vi "EINDE3.vi"() -> ()   [LabVIEW 2018]
uses:
  Kleuren- en afstandsensor/FSM States.ctl
  FSM States Project TOTAAL.ctl
panel:
  out "Achteruit":i32
  out "Timerrijden":i32
  out "Initial State":T1=enum."MOVE DOWNWARDS"
  out "Tussentijd":i32
  out "Timer":i32
  out "The End":bool
  in  "stop 3":bool
  in  "ON/OFF Grijper":bool
  in  "stop":bool
  in  "Aantal Witte blokjes":dbl
  in  "Aantal rode blokjes":dbl
  in  "Aantal Zwarte blokjes":dbl
  in  "LED aansturen":bool[](array[boolean])
  out "Current State":T1
  out "Motor":bool[](array[boolean])
  out "State to recover from":T1=enum."Stilstaan"
  in  "EMERGENCY":bool
  in  "Teller wit":dbl
  in  "Teller Rood":dbl
  in  "Teller zwart":dbl
  out "Wit":bool
  out "Zwart":bool
  out "Rood":bool
  in  "Kleurmaken":bool
  out "Kleuren veranderen":T2
  out "Analoge in":dbl[](array[numeric]) format="%0.2f"
  out "Afstand":bool
  # "INPUT"
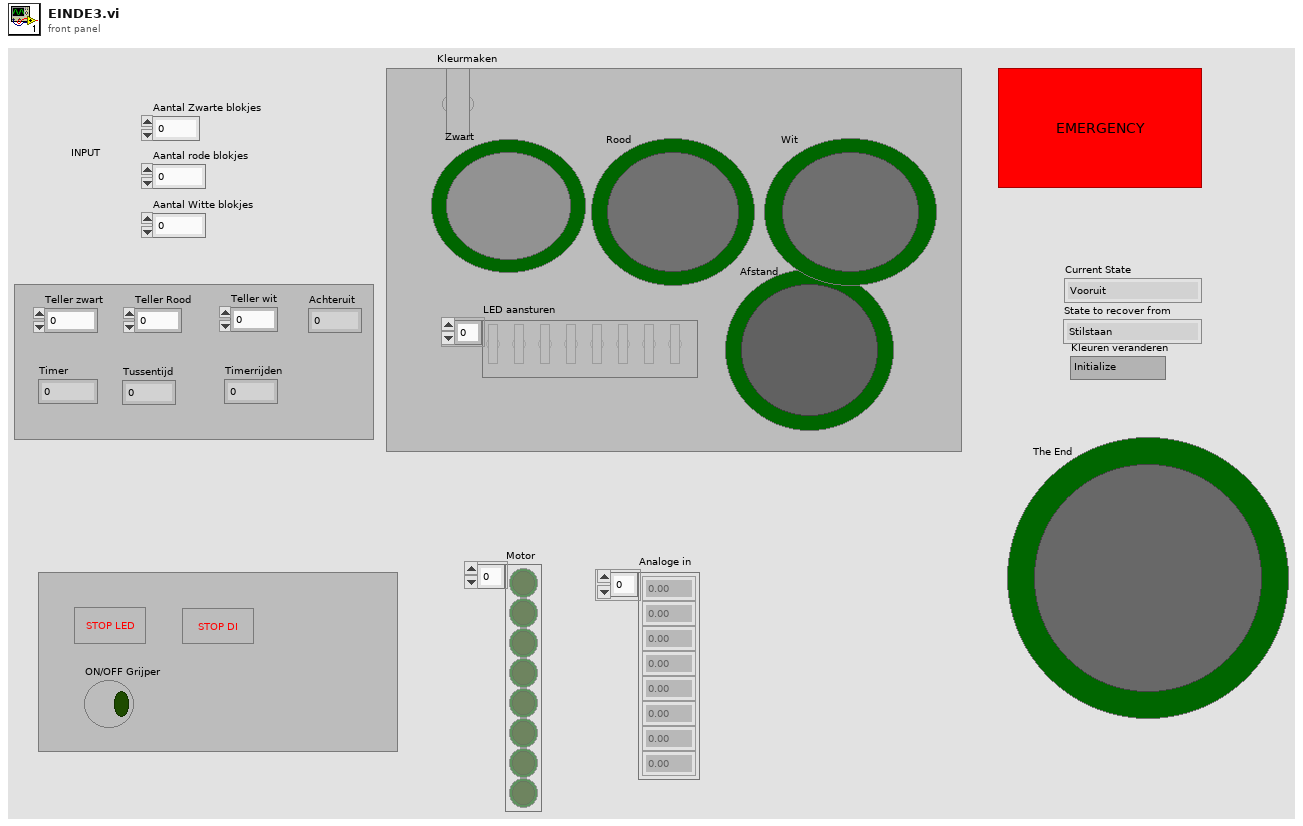
[diagram p1: front panel]
types:
  T1 = typedef "FSM States Project TOTAAL.ctl" = enum16{"Vooruit", "Achteruit", "Stilstaan", "EMERGENCY", "MOVE DOWNWARDS", "GRAB", "MOVE UPWARDS", "ROTATE", "DROP", "RETURN", "Stop "}
  T2 = typedef "FSM States.ctl" = enum16{"Initialize", "ROOD", "GROEN ", "Blauw "}
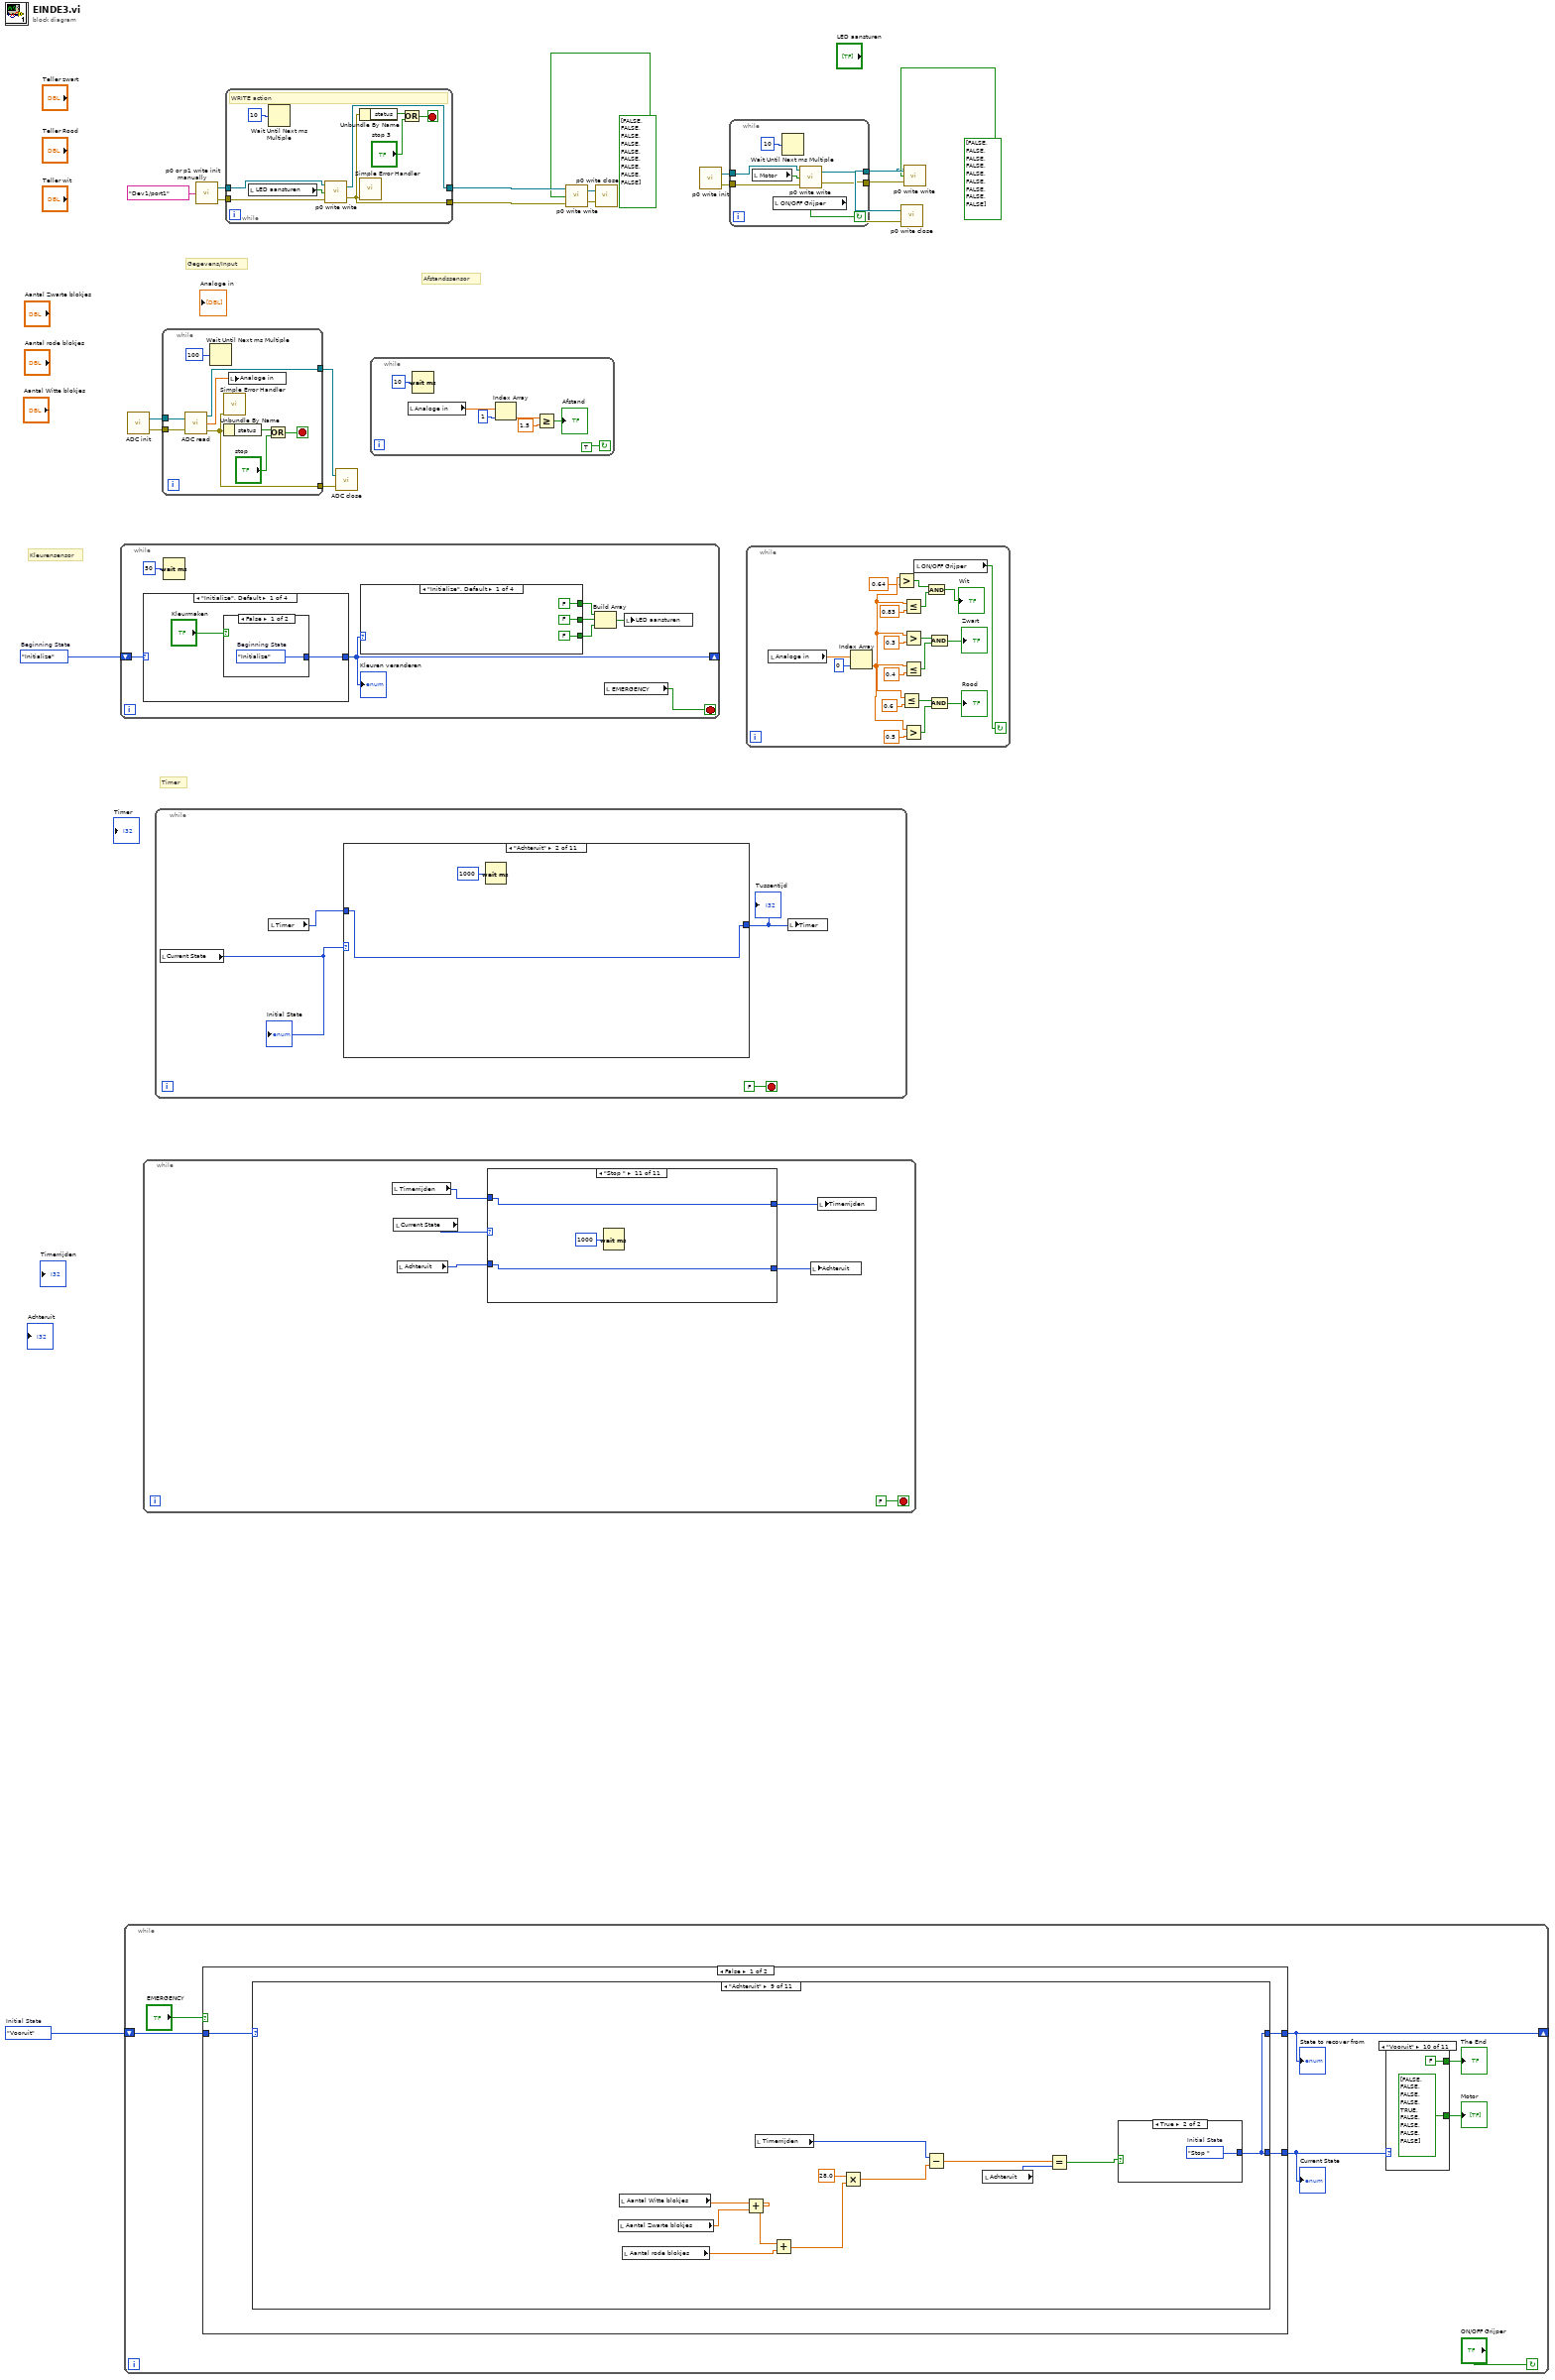
[diagram p0: block diagram]
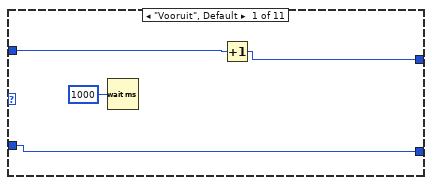
[diagram p2: hidden frame]
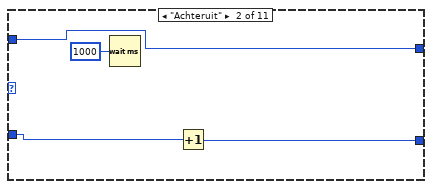
[diagram p3: hidden frame]
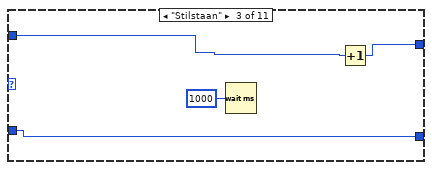
[diagram p4: hidden frame]
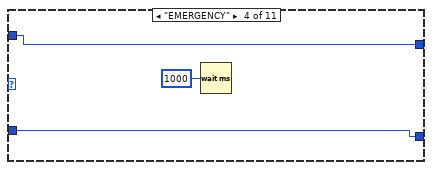
[diagram p5: hidden frame]
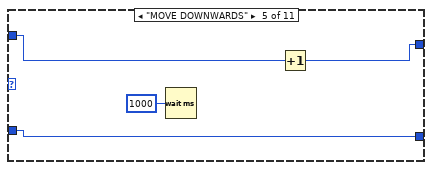
[diagram p6: hidden frame]
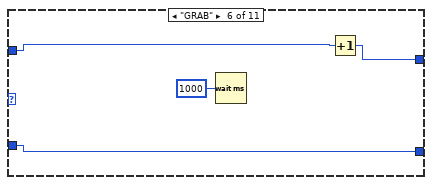
[diagram p7: hidden frame]
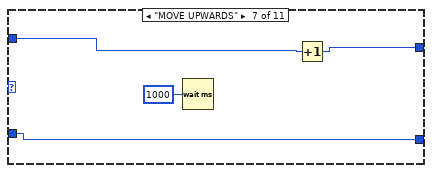
[diagram p8: hidden frame]
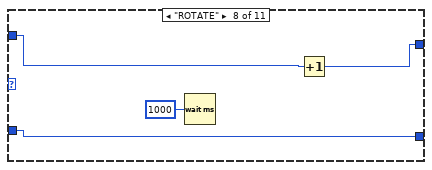
[diagram p9: hidden frame]
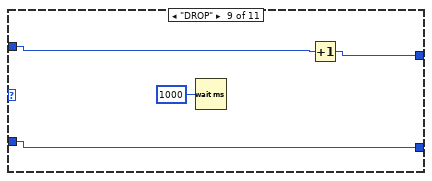
[diagram p10: hidden frame]
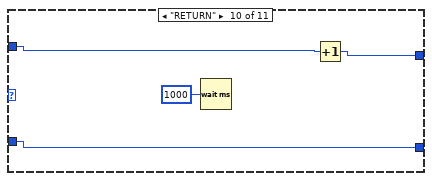
[diagram p11: hidden frame]
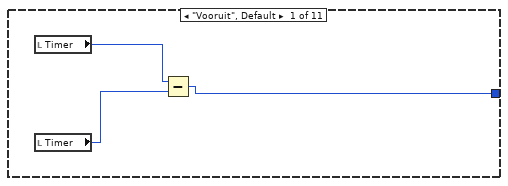
[diagram p12: hidden frame]
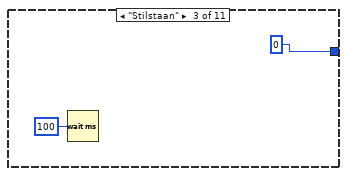
[diagram p13: hidden frame]
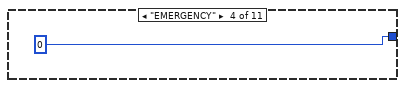
[diagram p14: hidden frame]
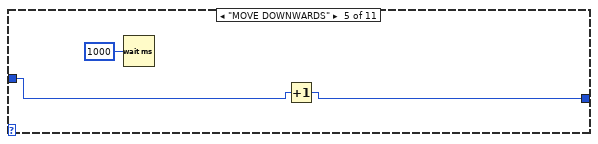
[diagram p15: hidden frame]
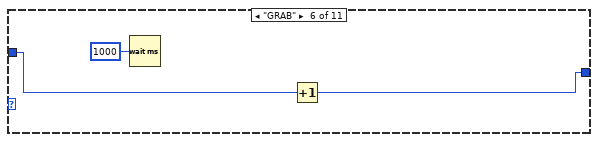
[diagram p16: hidden frame]
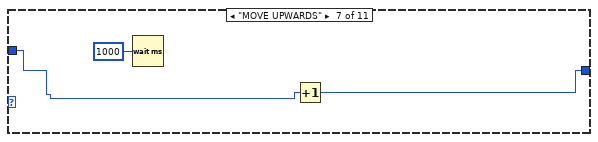
[diagram p17: hidden frame]
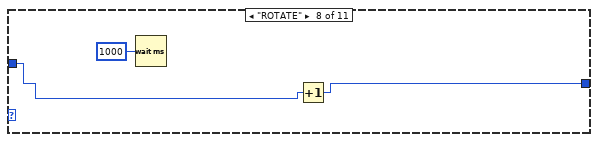
[diagram p18: hidden frame]
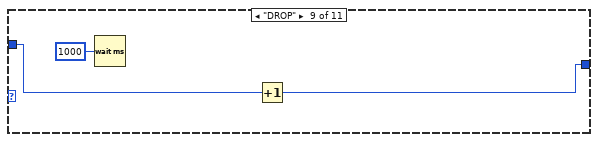
[diagram p19: hidden frame]
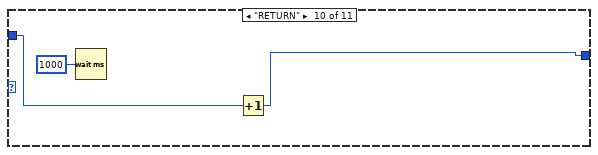
[diagram p20: hidden frame]
diagram:
  w1 = FSM_States_Project_TOTAAL."Vooruit"  # Initial State
  w17 = FSM_States."Initialize"  # Beginning State
  # "Timer"
  # "Gegevens/Input"
  # "Kleurensensor"
  # "Afstandssensor"
  n1 = while {
    shift-right: [w23] -> _
    shift-left: w17 -> [w29]
    stop <- w22 stop-if-true
    n2 = case shown="\"Initialize\", Default" w29 {
      tunnel: [w43 w46 w47 w48] -> w23
      frame "Initialize", Default {
        n3 = case shown="False" "Kleurmaken" {
          tunnel: [w44 w45] -> w43
          frame False {
            w44 = FSM_States."Initialize"  # Beginning State
          }
          frame True {
            w45 = FSM_States."ROOD"  # Beginning State
          }
        }
      }
      frame "ROOD" {
        w46 = FSM_States."GROEN "  # Beginning State
      }
      frame "GROEN " {
        w47 = FSM_States."Blauw "  # Beginning State
      }
      frame "Blauw " {
        w48 = FSM_States."ROOD"  # Beginning State
      }
    }
    "Kleuren veranderen" <- w23
    n4 = Wait (ms)(milliseconds to wait=u32 50) -> ()  [unwired: 1 out]
    n5 = case shown="\"Initialize\", Default" w23 {
      tunnel: [FALSE FALSE FALSE TRUE] -> w26
      tunnel: [FALSE TRUE FALSE FALSE] -> w25
      tunnel: [FALSE FALSE TRUE FALSE] -> w24
      frame "Initialize", Default {
      }
      frame "ROOD" {
      }
      frame "GROEN " {
      }
      frame "Blauw " {
      }
    }
    n6 = Build Array(w26, w25, w24) -> (w27:bool[])
    n7 = local read "EMERGENCY"() -> (w22:bool)
    n8 = local write "LED aansturen"(w27) -> ()
  }
  n9 = while {
    shift-right: [w52] -> _
    shift-left: w1 -> [w53]
    stop <- "ON/OFF Grijper" continue-if-true
    n10 = case shown="False" "EMERGENCY" {
      tunnel: w53 -> [w80 _]
      tunnel: [w79 FSM_States_Project_TOTAAL."EMERGENCY" ("State to Recover from 2")] -> w51
      tunnel: [w78 w203] -> w52
      frame False {
        n11 = case shown="\"Achteruit\"" w80 {
          tunnel: [w81 w82 w88 w94 w100 w106 w112 w123 w195 w198 w202] -> w79
          tunnel: [w81 w82 w88 w94 w100 w106 w112 w123 w195 w198 w202] -> w78
          frame "EMERGENCY" {
            n12 = local read "State to recover from"() -> (w81:T1)
          }
          frame "MOVE DOWNWARDS" {
            n13 = local read "Timer"() -> (w85:i32)
            n14 = Greater Or Equal?(x=w85, y=8) -> (x >= y?=w83:bool)
            n15 = case shown="False" w83 {
              tunnel: [FSM_States_Project_TOTAAL."MOVE DOWNWARDS" FSM_States_Project_TOTAAL."GRAB"] -> w82
              frame False {
              }
              frame True {
              }
            }
          }
          frame "GRAB" {
            n16 = local read "Timer"() -> (w90:i32)
            n17 = Greater Or Equal?(x=w90, y=10) -> (x >= y?=w91:bool)
            n18 = case shown="True" w91 {
              tunnel: [w92 w93] -> w88
              frame False {
                w92 = FSM_States_Project_TOTAAL."GRAB"  # Next State
              }
              frame True {
                w93 = FSM_States_Project_TOTAAL."MOVE UPWARDS"  # Next State
              }
            }
          }
          frame "MOVE UPWARDS" {
            n19 = local read "Timer"() -> (w97:i32)
            n20 = Greater Or Equal?(x=w97, y=20) -> (x >= y?=w95:bool)
            n21 = case shown="True" w95 {
              tunnel: [w98 w99] -> w94
              frame False {
                w98 = FSM_States_Project_TOTAAL."MOVE UPWARDS"  # Next State
              }
              frame True {
                w99 = FSM_States_Project_TOTAAL."ROTATE"  # Next State
              }
            }
          }
          frame "ROTATE" {
            n22 = local read "Timer"() -> (w103:i32)
            n23 = Greater Or Equal?(x=w103, y=23) -> (x >= y?=w101:bool)
            n24 = case shown="False" w101 {
              tunnel: [w104 w105] -> w100
              frame False {
                w104 = FSM_States_Project_TOTAAL."ROTATE"  # Next State
              }
              frame True {
                w105 = FSM_States_Project_TOTAAL."DROP"  # Next State
              }
            }
          }
          frame "DROP" {
            n25 = local read "Timer"() -> (w109:i32)
            n26 = Greater Or Equal?(x=w109, y=25) -> (x >= y?=w107:bool)
            n27 = case shown="True" w107 {
              tunnel: [w110 w111] -> w106
              frame False {
                w110 = FSM_States_Project_TOTAAL."DROP"  # Next State
              }
              frame True {
                w111 = FSM_States_Project_TOTAAL."RETURN"  # Next State
              }
            }
          }
          frame "RETURN" {
            n28 = local read "Timer"() -> (w114:i32)
            n29 = Greater Or Equal?(x=w114, y=28) -> (x >= y?=w115:bool)
            n30 = case shown="True" w115 {
              tunnel: [w116 w117] -> w112
              frame False {
                w116 = FSM_States_Project_TOTAAL."RETURN"  # Next State
              }
              frame True {
                w117 = FSM_States_Project_TOTAAL."Vooruit"  # Next State
              }
            }
          }
          frame "Stilstaan" {
            n31 = local read "Afstand"() -> (w122:bool)
            n32 = Wait (ms)(milliseconds to wait=u32 10) -> ()  [unwired: 1 out]
            n33 = local read "Zwart"() -> (w120:bool)
            n34 = local read "Rood"() -> (w121:bool)
            n35 = local read "Wit"() -> (w119:bool)
            n36 = case shown="True" w122 {
              tunnel: [w124 w128] -> w123
              tunnel: w121 -> [_ w127]
              tunnel: w120 -> [_ w126]
              tunnel: w119 -> [_ w125]
              frame False {
                w124 = FSM_States_Project_TOTAAL."Vooruit"  # Initial State
              }
              frame True {
                n37 = case shown="False" w127 {
                  tunnel: [w131 w179] -> w128
                  tunnel: w126 -> [w130 _]
                  tunnel: w125 -> [w129 _]
                  frame False {
                    n38 = case shown="True" w130 {
                      tunnel: [w133 w169] -> w131
                      tunnel: w129 -> [w132 _]
                      frame False {
                        n39 = case shown="True" w132 {
                          tunnel: [w134 w140] -> w133
                          frame False {
                            w134 = FSM_States_Project_TOTAAL."Stilstaan"  # Initial State
                          }
                          frame True {
                            n40 = local read "Aantal Witte blokjes"() -> (w137:dbl)
                            n41 = local read "Teller wit"() -> (w138:dbl)
                            n42 = Subtract(x=w137, y=w138) -> (x-y=w139:dbl)
                            n43 = Not Equal?(x=w139, y=0.0) -> (x != y?=w135:bool)
                            n44 = case shown="False" w135 {
                              tunnel: [w141 w161] -> w140
                              frame False {
                                n45 = local read "Aantal rode blokjes"() -> (w158:dbl)
                                n46 = local read "Aantal Zwarte blokjes"() -> (w154:dbl)
                                n47 = local read "Teller zwart"() -> (w153:dbl)
                                n48 = local read "Aantal Witte blokjes"() -> (w149:dbl)
                                n49 = local read "Teller Rood"() -> (w157:dbl)
                                n50 = local read "Teller wit"() -> (w148:dbl)
                                n51 = Subtract(x=w149, y=w148) -> (x-y=w147:dbl)
                                n52 = Subtract(x=w158, y=w157) -> (x-y=w156:dbl)
                                n53 = Subtract(x=w154, y=w153) -> (x-y=w152:dbl)
                                n54 = Not Equal?(x=w156, y=0.0) -> (x != y?=w146:bool)
                                n55 = Not Equal?(x=w152, y=0.0) -> (x != y?=w145:bool)
                                n56 = Not Equal?(x=w147, y=0.0) -> (x != y?=w144:bool)
                                n57 = Or(x=w146, y=w145) -> (x .or. y?=w143:bool)
                                n58 = Or(x=w143, y=w144) -> (x .or. y?=w142:bool)
                                n59 = case shown="False" w142 {
                                tunnel: [w159 w160] -> w141
                                frame False {
                                w159 = FSM_States_Project_TOTAAL."Achteruit"  # Initial State
                                }
                                frame True {
                                w160 = FSM_States_Project_TOTAAL."Vooruit"  # Initial State
                                }
                                }
                              }
                              frame True {
                                w161 = FSM_States_Project_TOTAAL."MOVE DOWNWARDS"  # Initial State
                                n60 = local read "Teller wit"() -> (w163:dbl)
                                n61 = Increment(x=w163) -> (x+1=w162:dbl)
                                n62 = local write "Teller wit"(w162) -> ()
                              }
                            }
                          }
                        }
                      }
                      frame True {
                        n63 = local read "Aantal Zwarte blokjes"() -> (w167:dbl)
                        n64 = local read "Teller zwart"() -> (w168:dbl)
                        n65 = Subtract(x=w167, y=w168) -> (x-y=w165:dbl)
                        n66 = Not Equal?(x=w165, y=0.0) -> (x != y?=w164:bool)
                        n67 = case shown="False" w164 {
                          tunnel: [w170 w171] -> w169
                          frame False {
                            w170 = FSM_States_Project_TOTAAL."Vooruit"  # Initial State
                          }
                          frame True {
                            w171 = FSM_States_Project_TOTAAL."MOVE DOWNWARDS"  # Initial State
                            n68 = local read "Teller zwart"() -> (w173:dbl)
                            n69 = Increment(x=w173) -> (x+1=w172:dbl)
                            n70 = local write "Teller zwart"(w172) -> ()
                          }
                        }
                      }
                    }
                  }
                  frame True {
                    n71 = local read "Aantal rode blokjes"() -> (w178:dbl)
                    n72 = local read "Teller Rood"() -> (w177:dbl)
                    n73 = Subtract(x=w178, y=w177) -> (x-y=w175:dbl)
                    n74 = Not Equal?(x=w175, y=0.0) -> (x != y?=w174:bool)
                    n75 = case shown="False" w174 {
                      tunnel: [w180 w183] -> w179
                      frame False {
                        w180 = FSM_States_Project_TOTAAL."Vooruit"  # Initial State
                      }
                      frame True {
                        w183 = FSM_States_Project_TOTAAL."MOVE DOWNWARDS"  # Initial State
                        n76 = local read "Teller Rood"() -> (w182:dbl)
                        n77 = Increment(x=w182) -> (x+1=w181:dbl)
                        n78 = local write "Teller Rood"(w181) -> ()
                      }
                    }
                  }
                }
              }
            }
          }
          frame "Achteruit" {
            n79 = local read "Aantal Zwarte blokjes"() -> (w192:dbl)
            n80 = local read "Aantal Witte blokjes"() -> (w193:dbl)
            n81 = local read "Aantal rode blokjes"() -> (w190:dbl)
            n82 = Add(x=w193, y=w192) -> (x+y=w191:dbl)
            n83 = local read "Timerrijden"() -> (w187:i32)
            n84 = Add(x=w191, y=w190) -> (x+y=w189:dbl)
            n85 = Multiply(x=28.0, y=w189) -> (x*y=w186:dbl)
            n86 = Subtract(x=w187, y=w186) -> (x-y=w185:dbl)
            n87 = local read "Achteruit"() -> (w184:i32)
            n88 = Equal?(x=w185, y=w184) -> (x = y?=w194:bool)
            n89 = case shown="True" w194 {
              tunnel: [w196 w197] -> w195
              frame False {
                w196 = FSM_States_Project_TOTAAL."Achteruit"  # Initial State
              }
              frame True {
                w197 = FSM_States_Project_TOTAAL."Stop "  # Initial State
              }
            }
          }
          frame "Vooruit" {
            n90 = local read "Afstand"() -> (w199:bool)
            n91 = case shown="False" w199 {
              tunnel: [w200 w201] -> w198
              frame False {
                w200 = FSM_States_Project_TOTAAL."Vooruit"  # Initial State
              }
              frame True {
                w201 = FSM_States_Project_TOTAAL."Stilstaan"  # Initial State
              }
            }
          }
          frame "Stop " {
            w202 = FSM_States_Project_TOTAAL."Stop "  # Initial State
          }
        }
      }
      frame True {
        n92 = local read "State to recover from"() -> (w203:T1)
      }
    }
    "State to recover from" <- w52
    "Current State" <- w51
    n93 = case shown="\"Vooruit\"" w51 {
      tunnel: [bool[] [FALSE, FALSE, FALSE, FALSE, FALSE, FALSE, FALSE, FALSE, FALSE] ("digital out") bool[] [FALSE, FALSE, TRUE, FALSE, FALSE, FALSE, FALSE, FALSE, FALSE] ("digital out") bool[] [FALSE, FALSE, FALSE, FALSE, FALSE, FALSE, TRUE, FALSE, FALSE] ("digital out") bool[] [FALSE, FALSE, FALSE, TRUE, FALSE, FALSE, FALSE, FALSE, FALSE] ("digital out") bool[] [TRUE, FALSE, FALSE, FALSE, FALSE, FALSE, FALSE, FALSE, FALSE] ("digital out") bool[] [FALSE, FALSE, FALSE, FALSE, FALSE, FALSE, FALSE, TRUE, FALSE] ("digital out") bool[] [FALSE, TRUE, FALSE, FALSE, FALSE, FALSE, FALSE, FALSE, FALSE] ("digital out") bool[] [FALSE, FALSE, FALSE, FALSE, FALSE, FALSE, FALSE, FALSE, FALSE] ("digital out") bool[] [FALSE, FALSE, FALSE, FALSE, FALSE, TRUE, FALSE, FALSE, FALSE] ("digital out") bool[] [FALSE, FALSE, FALSE, FALSE, TRUE, FALSE, FALSE, FALSE, FALSE] ("digital out") bool[] [FALSE, FALSE, FALSE, FALSE, FALSE, FALSE, FALSE, FALSE, FALSE] ("digital out")] -> w49
      tunnel: [FALSE ("The End") FALSE ("The End") FALSE ("The End") FALSE ("The End") FALSE ("The End") FALSE ("The End") FALSE ("The End") FALSE ("The End") FALSE ("The End") FALSE ("The End") TRUE ("The End")] -> w50
      frame "EMERGENCY" {
      }
      frame "MOVE DOWNWARDS" {
      }
      frame "GRAB" {
      }
      frame "MOVE UPWARDS" {
      }
      frame "ROTATE" {
      }
      frame "DROP" {
      }
      frame "RETURN" {
      }
      frame "Stilstaan" {
      }
      frame "Achteruit" {
      }
      frame "Vooruit" {
      }
      frame "Stop " {
      }
    }
    "Motor" <- w49
    "The End" <- w50
  }
  n94 = call "ADC init.vi"() -> ("error out"=w20:errorcluster, "task out"=w21:refnum<k21>)
  n95 = while {
    stop <- FALSE stop-if-true
    n96 = local read "Timerrijden"() -> (w206:i32)
    n97 = local read "Current State"() -> (w209:T1)
    n98 = local read "Achteruit"() -> (w208:i32)
    n99 = case shown="\"Stop \"" w209 {
      tunnel: w208 -> [w214 w218 w220 w223 w226 w231 w234 w238 w242 w246 w251]
      tunnel: [w214 w217 w220 w223 w226 w231 w234 w238 w242 w246 w251] -> w207
      tunnel: w206 -> [w213 w215 w219 w224 w227 w230 w235 w240 w243 w247 w250]
      tunnel: [w212 w215 w221 w224 w228 w232 w236 w239 w244 w248 w250] -> w205
      frame "Vooruit", Default {
        n100 = Wait (ms)(milliseconds to wait=u32 1000) -> ()  [unwired: 1 out]
        n101 = Increment(x=w213) -> (x+1=w212:i32)
      }
      frame "Achteruit" {
        n102 = Wait (ms)(milliseconds to wait=u32 1000) -> ()  [unwired: 1 out]
        n103 = Increment(x=w218) -> (x+1=w217:i32)
      }
      frame "Stilstaan" {
        n104 = Wait (ms)(milliseconds to wait=u32 1000) -> ()  [unwired: 1 out]
        n105 = Increment(x=w219) -> (x+1=w221:i32)
      }
      frame "EMERGENCY" {
        n106 = Wait (ms)(milliseconds to wait=u32 1000) -> ()  [unwired: 1 out]
      }
      frame "MOVE DOWNWARDS" {
        n107 = Wait (ms)(milliseconds to wait=u32 1000) -> ()  [unwired: 1 out]
        n108 = Increment(x=w227) -> (x+1=w228:i32)
      }
      frame "GRAB" {
        n109 = Wait (ms)(milliseconds to wait=u32 1000) -> ()  [unwired: 1 out]
        n110 = Increment(x=w230) -> (x+1=w232:i32)
      }
      frame "MOVE UPWARDS" {
        n111 = Wait (ms)(milliseconds to wait=u32 1000) -> ()  [unwired: 1 out]
        n112 = Increment(x=w235) -> (x+1=w236:i32)
      }
      frame "ROTATE" {
        n113 = Wait (ms)(milliseconds to wait=u32 1000) -> ()  [unwired: 1 out]
        n114 = Increment(x=w240) -> (x+1=w239:i32)
      }
      frame "DROP" {
        n115 = Wait (ms)(milliseconds to wait=u32 1000) -> ()  [unwired: 1 out]
        n116 = Increment(x=w243) -> (x+1=w244:i32)
      }
      frame "RETURN" {
        n117 = Wait (ms)(milliseconds to wait=u32 1000) -> ()  [unwired: 1 out]
        n118 = Increment(x=w247) -> (x+1=w248:i32)
      }
      frame "Stop " {
        n119 = Wait (ms)(milliseconds to wait=u32 1000) -> ()  [unwired: 1 out]
      }
    }
    n120 = local write "Achteruit"(w207) -> ()
    n121 = local write "Timerrijden"(w205) -> ()
  }
  n122 = while {
    stop <- FALSE stop-if-true
    n123 = local read "Current State"() -> (w253:T1)
    "Initial State" <- w253
    n124 = local read "Timer"() -> (w255:i32)
    n125 = case shown="\"Achteruit\"" w253 {
      tunnel: w255 -> [_ w260 _ _ w266 w269 w272 w275 w278 w281 _]
      tunnel: [w259 w260 0 ("Timer2") 0 ("Timer2") w265 w268 w271 w274 w277 w280 0 ("Timer2")] -> w254
      frame "Vooruit", Default {
        n126 = local read "Timer"() -> (w257:i32)
        n127 = local read "Timer"() -> (w258:i32)
        n128 = Subtract(x=w257, y=w258) -> (x-y=w259:i32)
      }
      frame "Achteruit" {
        n129 = Wait (ms)(milliseconds to wait=u32 1000) -> ()  [unwired: 1 out]
      }
      frame "Stilstaan" {
        n130 = Wait (ms)(milliseconds to wait=u32 100) -> ()  [unwired: 1 out]
      }
      frame "EMERGENCY" {
      }
      frame "MOVE DOWNWARDS" {
        n131 = Wait (ms)(milliseconds to wait=u32 1000) -> ()  [unwired: 1 out]
        n132 = Increment(x=w266) -> (x+1=w265:i32)
      }
      frame "GRAB" {
        n133 = Wait (ms)(milliseconds to wait=u32 1000) -> ()  [unwired: 1 out]
        n134 = Increment(x=w269) -> (x+1=w268:i32)
      }
      frame "MOVE UPWARDS" {
        n135 = Wait (ms)(milliseconds to wait=u32 1000) -> ()  [unwired: 1 out]
        n136 = Increment(x=w272) -> (x+1=w271:i32)
      }
      frame "ROTATE" {
        n137 = Wait (ms)(milliseconds to wait=u32 1000) -> ()  [unwired: 1 out]
        n138 = Increment(x=w275) -> (x+1=w274:i32)
      }
      frame "DROP" {
        n139 = Wait (ms)(milliseconds to wait=u32 1000) -> ()  [unwired: 1 out]
        n140 = Increment(x=w278) -> (x+1=w277:i32)
      }
      frame "RETURN" {
        n141 = Wait (ms)(milliseconds to wait=u32 1000) -> ()  [unwired: 1 out]
        n142 = Increment(x=w281) -> (x+1=w280:i32)
      }
      frame "Stop " {
      }
    }
    "Tussentijd" <- w254
    n143 = local write "Timer"(w254) -> ()
  }
  n144 = while {
    tunnel: w21 -> [w292]
    tunnel: w20 -> [w291]
    tunnel: [w288] -> w19
    tunnel: [w290] -> w18
    stop <- w285 stop-if-true
    n145 = call "ADC read.vi"("task/channels in"=w292, "error in"=w291) -> ("task out"=w290:refnum<k21>, "analog in"=w284:dbl[], "error out"=w288:errorcluster)
    n146 = Wait Until Next ms Multiple(millisecond multiple=u32 100) -> ()  [unwired: 1 out]
    n147 = call <vilib>:"Simple Error Handler.vi"("error in (no error)"=w288) -> ()  [unwired: 4 in, 5 out]
    n148 = Unbundle By Name(w288) -> ("status"=w287:bool)
    n149 = local write "Analoge in"(w284) -> ()
    n150 = Or(x=w287, y="stop") -> (x .or. y?=w285:bool)
  }
  n151 = call "p0 or p1 write init manually.vi"("Port"=tag "Dev1/port1") -> ("task out"=w11:refnum<k21>, "error out"=w10:errorcluster)
  n152 = while {
    tunnel: w11 -> [w301]
    tunnel: [w300] -> w16
    tunnel: w10 -> [w299]
    tunnel: [w295] -> w15
    stop <- w296 stop-if-true
    # "WRITE action"
    n153 = local read "LED aansturen"() -> (w293:bool[])
    n154 = Wait Until Next ms Multiple(millisecond multiple=u32 10) -> ()  [unwired: 1 out]
    n155 = call "p0 write write.vi"("error in"=w299, "digital out"=w293, "task/channels in"=w301) -> ("error out"=w295:errorcluster, "task out"=w300:refnum<k21>)
    n156 = Unbundle By Name(w295) -> ("status"=w294:bool)
    n157 = call <vilib>:"Simple Error Handler.vi"("error in (no error)"=w295) -> ()  [unwired: 4 in, 5 out]
    n158 = Or(x=w294, y="stop 3") -> (x .or. y?=w296:bool)
  }
  n159 = call "ADC close.vi"("error in"=w19, "task/channels in"=w18) -> ()
  n160 = while {
    stop <- TRUE continue-if-true
    n161 = local read "Analoge in"() -> (w302:dbl[])
    n162 = Wait (ms)(milliseconds to wait=u32 10) -> ()  [unwired: 1 out]
    n163 = Index Array(array=w302, index=1) -> (element=w306:dbl)
    n164 = Greater Or Equal?(x=w306, y=1.5) -> (x >= y?=→"Afstand":bool)
  }
  n165 = call "p0 write write.vi"("error in"=w15, "digital out"=bool[] [FALSE, FALSE, FALSE, FALSE, FALSE, FALSE, FALSE, FALSE, FALSE], "task/channels in"=w16) -> ("error out"=w13:errorcluster, "task out"=w14:refnum<k21>)
  n166 = call "p0 write close.vi"("error in"=w13, "task/channels in"=w14) -> ()
  n167 = call "p0 write init.vi"() -> ("error out"=w3:errorcluster, "task out"=w2:refnum<k21>)
  n168 = while {
    tunnel: [w314] -> w5
    tunnel: [w313] -> w4
    tunnel: w3 -> [w311]
    tunnel: w2 -> [w312]
    stop <- w315 continue-if-true
    n169 = local read "Motor"() -> (w309:bool[])
    n170 = local read "ON/OFF Grijper"() -> (w315:bool)
    n171 = Wait Until Next ms Multiple(millisecond multiple=u32 10) -> ()  [unwired: 1 out]
    n172 = call "p0 write write.vi"("error in"=w311, "digital out"=w309, "task/channels in"=w312) -> ("error out"=w314:errorcluster, "task out"=w313:refnum<k21>)
  }
  n173 = while {
    stop <- w321 continue-if-true
    n174 = local read "Analoge in"() -> (w333:dbl[])
    n175 = Index Array(array=w333, index=0) -> (element=w317:dbl)
    n176 = Greater?(x=w317, y=0.64) -> (0:w318:bool)
    n177 = Less Or Equal?(x=w317, y=0.6) -> (x <= y?=w323:bool)
    n178 = Less Or Equal?(x=w317, y=0.83) -> (x <= y?=w320:bool)
    n179 = Greater?(x=w317, y=0.3) -> (0:w329:bool)
    n180 = Less Or Equal?(x=w317, y=0.4) -> (x <= y?=w328:bool)
    n181 = Greater?(x=w317, y=0.5) -> (0:w322:bool)
    n182 = local read "ON/OFF Grijper"() -> (w321:bool)
    n183 = And(x=w318, y=w320) -> (x .and. y?=→"Wit":bool)
    n184 = And(x=w329, y=w328) -> (x .and. y?=→"Zwart":bool)
    n185 = And(x=w323, y=w322) -> (x .and. y?=→"Rood":bool)
  }
  n186 = call "p0 write write.vi"("error in"=w5, "digital out"=bool[] [FALSE, FALSE, FALSE, FALSE, FALSE, FALSE, FALSE, FALSE, FALSE], "task/channels in"=w4) -> ("error out"=w7:errorcluster, "task out"=w8:refnum<k21>)
  n187 = call "p0 write close.vi"("error in"=w7, "task/channels in"=w8) -> ()
